vi "Del AOI from list.vi"(1 "Coordinates of  AOI to delete":u16[](array[numeric])) -> (0 "Number of AOIs":i32)   [LabVIEW 2011]
doc: "Delete the AOI in the AOI list which is closest to the x and y coordinates given."
uses:
  AOI List Globals.vi
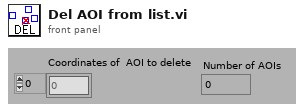
[diagram p1: front panel]
types:
  T1 = cluster{"AOI List[0]":u16, "AOI List[1]":u16, "AOI List[2]":u16, "AOI List[3]":u16}
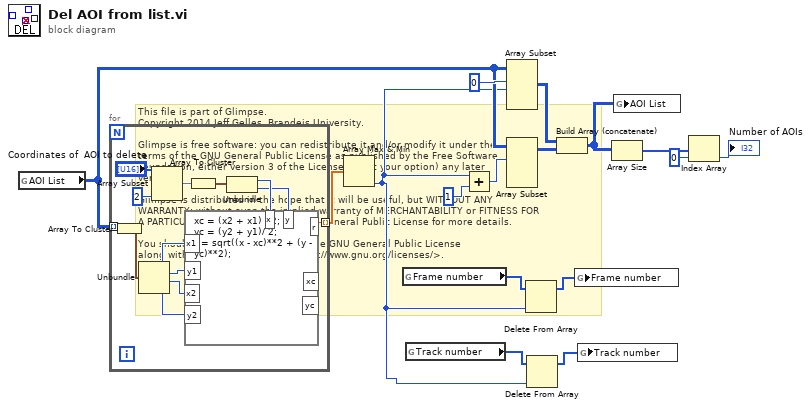
[diagram p0: block diagram]
diagram:
  # "This file is part of Glimpse. \nCopyright 2014 Jeff Gelles, Brandeis University.    \n\nGlimpse is free software: you can redistribute it and/or modify it under the \nterms of the GNU General Public License as published by the Free Software \nFoundation, either version 3 of the License, or (at your option) any later \nversion.\n\nGlimpse is distributed in the hope that it will be useful, but WITHOUT ANY \nWARRANTY; without even the implied warranty of MERCHANTABILITY or FITNESS FOR \nA PARTICULAR PURPOSE.  See the GNU General Public License for more details.\n\nYou should have received a copy of the GNU General Public License\nalong with Glimpse.  If not, see <http://www.gnu.org/licenses/>."
  n1 = global read "AOI List Globals.vi" "AOI List"() -> (w7:u16[][])
  n2 = for {
    tunnel: [w23] -> w6 mode=indexing
    tunnel: w7 -> [w21] mode=indexing
    n3 = Array To Cluster(array=w21) -> (cluster=w24:T1)
    n4 = Unbundle(w24) -> ("AOI List[0]"=w20:u16, "AOI List[1]"=w17:u16, "AOI List[2]"=w18:u16, "AOI List[3]"=w19:u16)
    n5 = Array Subset(array="Coordinates of  AOI to delete", length=2) -> (w28:u16[])  [unwired: 1 in]
    n6 = Array To Cluster(array=w28) -> (cluster=w27:cluster{"[0]":u16, "[1]":u16})
    n7 = Unbundle(w27) -> ("[0]"=w26:u16, "[1]"=w25:u16)
    n8 = formula code="xc = (x2 + x1) / 2;\nyc = (y2 + y1)/ 2;\nr = sqrt((x - xc)**2 + (y - yc)**2);"("x"=w26, "y"=w25, "x1"=w20, "y1"=w17, "x2"=w18, "y2"=w19) -> ("r"=w23:dbl)  [unwired: 2 out]
  }
  n9 = Array Max & Min(array=w6) -> (min index (indices)=w1:i32)  [unwired: 3 out]
  n10 = global read "AOI List Globals.vi" "Frame number"() -> (w5:i32[])
  n11 = global read "AOI List Globals.vi" "Track number"() -> (w2:u16[])
  n12 = Add(x=w1, y=1) -> (x+y=w11:i32)
  n13 = Array Subset(array=w7, index (row)=0, length (row)=w1) -> (w15:u16[][])  [unwired: 2 in]
  n14 = Array Subset(array=w7, index (row)=w11) -> (w14:u16[][])  [unwired: 3 in]
  n15 = Delete From Array(array=w5, index=w1) -> (array with subset deleted=w4:i32[])  [unwired: 1 in, 1 out]
  n16 = Delete From Array(array=w2, index=w1) -> (array with subset deleted=w3:u16[])  [unwired: 1 in, 1 out]
  n17 = Build Array (concatenate)(w15, w14) -> (w10:u16[][])
  n18 = global write "AOI List Globals.vi" "Frame number"(w4) -> ()
  n19 = global write "AOI List Globals.vi" "Track number"(w3) -> ()
  n20 = Array Size(array=w10) -> (size(s)=w9:i32[])
  n21 = global write "AOI List Globals.vi" "AOI List"(w10) -> ()
  n22 = Index Array(array=w9, index=0) -> (element=→"Number of AOIs":i32)
